vi "MGI Export Image Dialog.vi"(8 "error in (no error)":errorcluster, 9 "Image Type":T2(radio), 10 "Default Location(\"\")":path, 11 "Image Data":T1) -> (0 "error out":errorcluster)   [LabVIEW 2020]
doc: "This VI displays a dialog that allows a user to save the \"Image Data\" image to disk.\n\nAuthored by Brandon D. Steele\nsupport@mooregoodideas.com\nwww.mooregoodideas.com\n\nCopyright (c) 2010, Moore Good Ideas, Inc.\n\nAll rights reserved.\n\nRedistribution and use in source and binary forms, with or without modification, are permitted provided that the following conditions are met:\n\n * Redistributions of source code must retain the above copyright notice, this list of conditions and the following disclaimer.\n * Redistributions in binary form must reproduce the above copyright notice, this list of conditions and the following disclaimer in the documentation and/or other materials provided with the distribution.\n * Neither the name of Moore Good Ideas, Inc. nor the names of its contributors may be used to endorse or promote products derived from this software without specific prior written permission.\n\nTHIS SOFTWARE IS PROVIDED BY THE COPYRIGHT HOLDERS AND CONTRIBUTORS \"AS IS\" AND ANY EXPRESS OR IMPLIED WARRANTIES, INCLUDING, BUT NOT LIMITED TO, THE IMPLIED WARRANTIES OF MERCHANTABILITY AND FITNESS FOR A PARTICULAR PURPOSE ARE DISCLAIMED. IN NO EVENT SHALL THE COPYRIGHT OWNER OR CONTRIBUTORS BE LIABLE FOR ANY DIRECT, INDIRECT, INCIDENTAL, SPECIAL, EXEMPLARY, OR CONSEQUENTIAL DAMAGES (INCLUDING, BUT NOT LIMITED TO, PROCUREMENT OF SUBSTITUTE GOODS OR SERVICES; LOSS OF USE, DATA, OR PROFITS; OR BUSINESS INTERRUPTION) HOWEVER CAUSED AND ON ANY THEORY OF LIABILITY, WHETHER IN CONTRACT, STRICT LIABILITY, OR TORT (INCLUDING NEGLIGENCE OR OTHERWISE) ARISING IN ANY WAY OUT OF THE USE OF THIS SOFTWARE, EVEN IF ADVISED OF THE POSSIBILITY OF SUCH DAMAGE."
uses:
  <vilib>/picture/picture.llb/imagedata.ctl
  <userlib>/_MGI/File/MGI Windows Folder Enum.ctl
panel:
  in  "Cancel":bool
  in  "Export":bool
  in  "Path":path
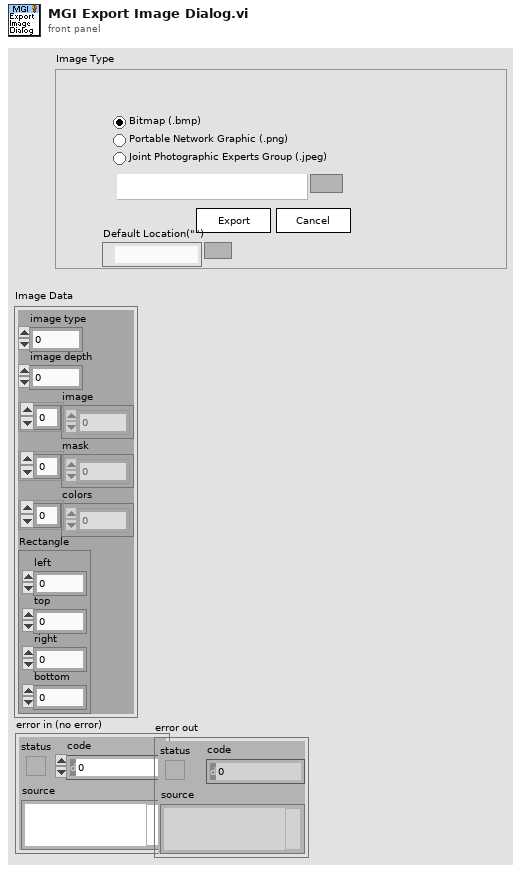
[diagram p1: front panel]
types:
  T1 = typedef "imagedata.ctl" = cluster{"image type":i32, "image depth":i32, "image":u8[], "mask":u8[], "colors":u32[], "Rectangle":cluster{"left":i16, "top":i16, "right":i16, "bottom":i16}}
  T2 = enum32{"Bitmap (.bmp)", "Portable Network Graphic (.png)", "Joint Photographic Experts Group (.jpeg)"}
  T3 = typedef "MGI Windows Folder Enum.ctl" = enum32{"Desktop", "Err<Internet>", "Programs", "Err<Controls>", "Err<Printers>", "Personal (MyDocuments)", "Favorites", "Startup", "Recent", "SendTo", "Err<RecycleBin>", "StartMenu", "Err<MyDocuments>", "MyMusic", "MyVideo", "Err<0x000F>", "DesktopDirectory", "Err<Drives>", "Err<Network>", "NetHood", "Fonts", "Templates", "CommonStartMenu", "CommonPrograms", "CommonStartup", "CommonDesktopDirectory", "AppData", "PrintHood", "LocalAppData", "Err<AltStartup>", "Err<CommonAltStartup>", "CommonFavorites", "InternetCache", "Cookies", "History", "CommonAppData", "Windows", "System", "ProgramFiles", "MyPictures", "Profile", "System32", "Err<0x002A>", "ProgramFilesCommon", "Err<0x002C>", "CommonTemplates", "CommonDocuments", "CommonAdminTools", "AdminTools"}
  T4 = cluster{"Prompt":string, "Match Pattern":string, "select mode":enum32{"existing file", "new file", "new or existing file", "existing dir", "new dir", "new or existing dir", "existing file (use LLBs)", "new file (use LLBs)", "new or existing file (use LLBs)", "new or existing file or directory (use LLBs)", "existing dir (use LLBs)", "new dir (use LLBs)", "new or existing dir (use LLBs)", "existing file or dir", "new file or dir", "new or existing file or dir", "existing file or dir (use LLBs)", "new file or dir (use LLBs)"}, "Start Path":path, "Pattern Label":string, "Button Text":string}
  T5 = enum8{"Enabled", "Disabled", "Disabled and Grayed Out"}
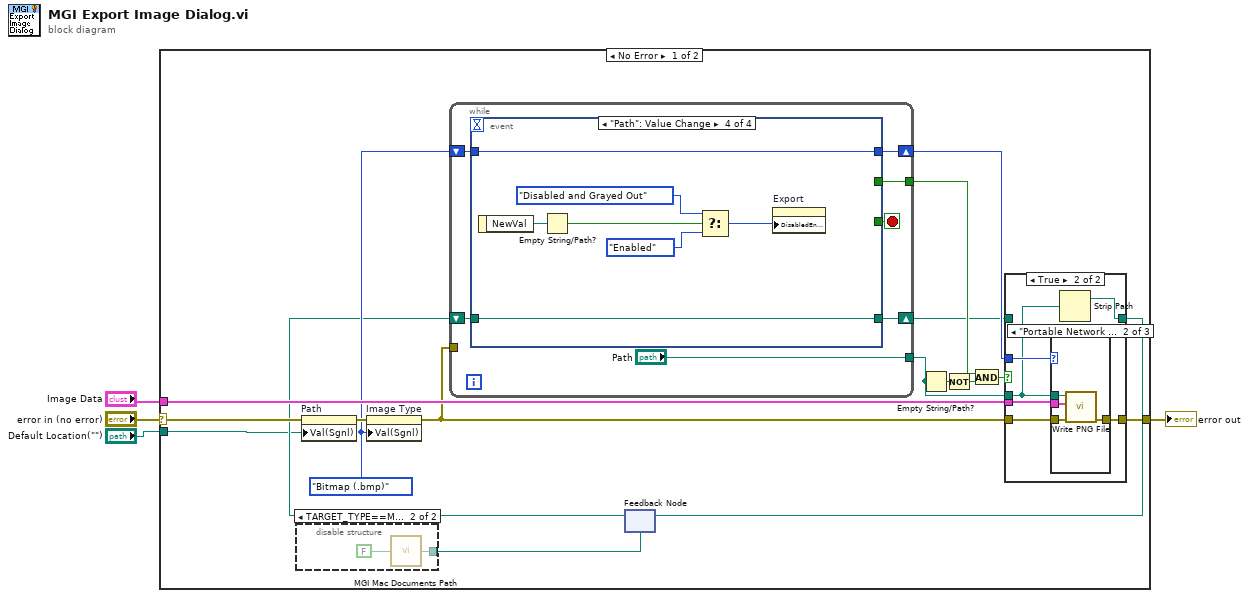
[diagram p0: block diagram]
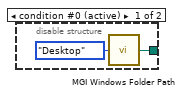
[diagram p2: hidden frame]
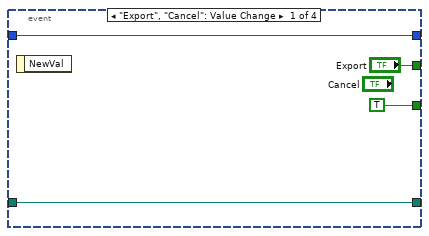
[diagram p3: hidden frame]
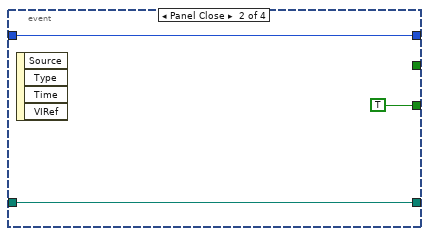
[diagram p4: hidden frame]
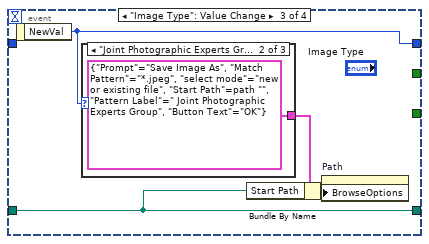
[diagram p5: hidden frame]
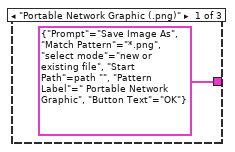
[diagram p6: hidden frame]
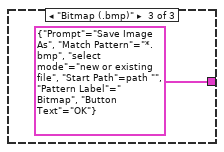
[diagram p7: hidden frame]
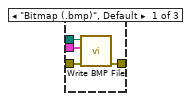
[diagram p9: hidden frame]
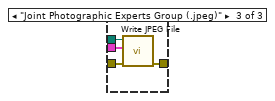
[diagram p10: hidden frame]
diagram:
  n1 = case shown="No Error" "error in (no error)" {
    selector: "error in (no error)" -> [w15 w74]
    tunnel: "Image Data" -> [w14 _]
    tunnel: [w12 w74] -> w2
    tunnel: "Default Location(\"\")" -> [w5 _]
    frame No Error {
      w11 = T2."Bitmap (.bmp)" ("Value (Signaling)")
      n2 = disable-structure shown="TARGET_TYPE==Mac" {
        disable-tunnel: [w22 w25] -> w9
        frame condition #0 (active) {
          n3 = call <userlib>:"MGI Windows Folder Path.vi"("Windows Folder"=MGI_Windows_Folder_Enum."Desktop" ("Special Folder")) -> ("Path"=w22:path)
        }
        frame condition #1 {
          n4 = call <userlib>:"MGI Mac Documents Path.vi"("User Documents? (F: Shared Documents)"=FALSE) -> ("Path"=w25:path)
        }
      }
      n5 = property on="Path" class="Path"(error in=w15, "Val(Sgnl)"=w5) -> (error out=w18:errorcluster)  [unwired: 1 in, 1 out]
      n6 = property on="Image Type" class="RadioBtnsControl (strict)"(error in=w18, "Val(Sgnl)"=w11) -> (error out=w13:errorcluster)  [unwired: 1 in, 1 out]
      n7 = feedback #1(w9) -> (w8:path)
      n8 = while {
        tunnel: [w32] -> w21
        tunnel: w13 -> [_]
        tunnel: ["Path"] -> w19
        shift-right: [w30] -> w10
        shift-left: w11 -> [w29]
        shift-right: [w27] -> w7
        shift-left: w8 -> [w28]
        stop <- w31 stop-if-true
        n9 = event shown="[3] \"Path\": Value Change" {
          selector: _ -> [_ _ _ _]
          dyn-events: _ -> [_ _ _ _]
          timeout: _ -> [_ _ _ _]
          tunnel: ["Export" _ _ _] -> w32
          tunnel: [TRUE TRUE _ _] -> w31
          tunnel: [w34 w38 w41 w51] -> w30
          tunnel: w29 -> [w34 w38 _ w51]
          tunnel: w28 -> [w33 w37 w40 w53]
          tunnel: [w33 w37 w40 w53] -> w27
          event "Export", "Cancel": Value Change {
            n10 = event-data() -> ()  [unwired: 2 out]
          }
          event Panel Close {
            n11 = event-data() -> ()  [unwired: 5 out]
          }
          event "Image Type": Value Change {
            n12 = event-data() -> ("NewVal"=w41:T2)  [unwired: 1 out]
            n13 = case shown="\"Joint Photographic Experts Group (.jpeg)\"" w41 {
              tunnel: [T4 {"Prompt"="Save Image As", "Match Pattern"="*.png", "select mode"=enum."new or existing file", "Start Path"=path "", "Pattern Label"=" Portable Network Graphic", "Button Text"="OK"} ("Browse Options") T4 {"Prompt"="Save Image As", "Match Pattern"="*.jpeg", "select mode"=enum."new or existing file", "Start Path"=path "", "Pattern Label"=" Joint Photographic Experts Group", "Button Text"="OK"} ("Browse Options") T4 {"Prompt"="Save Image As", "Match Pattern"="*.bmp", "select mode"=enum."new or existing file", "Start Path"=path "", "Pattern Label"=" Bitmap", "Button Text"="OK"} ("Browse Options")] -> w43
              frame "Portable Network Graphic (.png)" {
              }
              frame "Joint Photographic Experts Group (.jpeg)" {
              }
              frame "Bitmap (.bmp)" {
              }
            }
            n14 = Bundle By Name(cluster=w43, "Start Path"=w40) -> (w42:T4)
            n15 = property on="Path" class="Path"("BrowseOptions"=w42) -> ()  [unwired: 2 in, 2 out]
          }
          event "Path": Value Change {
            n16 = event-data() -> ("NewVal"=w52:path)  [unwired: 1 out]
            n17 = Empty String/Path?(string/path=w52) -> (empty?=w49:bool)
            n18 = Select(t=T5."Disabled and Grayed Out", s=w49, f=T5."Enabled" ("Disabled")) -> (s? t:f=w47:T5)
            n19 = property on="Export" class="Bool"("DisabledEnum"=w47) -> ()  [unwired: 2 in, 2 out]
          }
        }
      }
      n20 = Empty String/Path?(string/path=w19) -> (empty?=w17:bool)
      n21 = Not(x=w17) -> (.not. x?=w16:bool)
      n22 = And(x=w21, y=w16) -> (x .and. y?=w20:bool)
      n23 = case shown="True" w20 {
        tunnel: w10 -> [_ w61]
        tunnel: w14 -> [_ w60]
        tunnel: w19 -> [_ w57]
        tunnel: w13 -> [w55 w59]
        tunnel: [w55 w58] -> w12
        tunnel: w7 -> [w54 _]
        tunnel: [w54 w56] -> w6
        frame False {
        }
        frame True {
          n24 = case shown="\"Portable Network Graphic (.png)\"" w61 {
            tunnel: w60 -> [w64 w68 w72]
            tunnel: w57 -> [w65 w69 w73]
            tunnel: w59 -> [w62 w67 w70]
            tunnel: [w63 w66 w71] -> w58
            frame "Bitmap (.bmp)", Default {
              n25 = call <vilib>:"Write BMP File.vi"("error in (no error)"=w62, "image data"=w64, "path to BMP file"=w65) -> ("error out"=w63:errorcluster)  [unwired: 8 out]
            }
            frame "Portable Network Graphic (.png)" {
              n26 = call <vilib>:"Write PNG File.vi"("error in (no error)"=w67, "image data"=w68, "path to PNG file"=w69) -> ("error out"=w66:errorcluster)  [unwired: 8 out]
            }
            frame "Joint Photographic Experts Group (.jpeg)" {
              n27 = call <vilib>:"Write JPEG File.vi"("error in (no error)"=w70, "image data"=w72, "path to JPEG file"=w73) -> ("error out"=w71:errorcluster)  [unwired: 8 out]
            }
          }
          n28 = Strip Path(path=w57) -> (stripped path=w56:path)  [unwired: 1 out]
        }
      }
      n29 = feedback-in #1(w6) -> ()
    }
    frame Error {
    }
  }
  "error out" <- w2
